vi "Initialize.vi"(8 "error in (no error)":errorcluster, 11 "State in":T1={"State"=enum."Idle", "Start Time"=timestamp(0 s since 1904-01-01), "Current Time"=timestamp(0 s since 1904-01-01), "First Iteration"=FALSE, "Data"={"D-O State"=enum."Off"}, "Process Name"="", "Output Error"=FALSE, "Log Started"=FALSE, "Cycle Period"=50.0, "Configuration"={"Valve Settings"={"D-O Settings"={"DAQmx Task Name"="", "Output Channel"=0, "Output Channel Names"=[], "Run?"=FALSE}, "VICI Electronic Actuator"={"VISA resource name"="", "Mode"=enum."Two Positions With Stops", "Simulated"=FALSE}}, "Valve Type"=enum."Digital Output Valve", "Time On (Sec)"=0.0, "Time Off (Sec)"=0.0}} {"Configuration"."Valve Settings"."D-O Settings"."Output Channel" items=["Choose a Channel"]}) -> (0 "error out":errorcluster, 1 "Initialized":bool, 3 "State out":T1={"State"=enum."Idle", "Start Time"=timestamp(0 s since 1904-01-01), "Current Time"=timestamp(0 s since 1904-01-01), "First Iteration"=FALSE, "Data"={"D-O State"=enum."Off"}, "Process Name"="", "Output Error"=FALSE, "Log Started"=FALSE, "Cycle Period"=50.0, "Configuration"={"Valve Settings"={"D-O Settings"={"DAQmx Task Name"="", "Output Channel"=0, "Output Channel Names"=[], "Run?"=FALSE}, "VICI Electronic Actuator"={"VISA resource name"="", "Mode"=enum."Two Positions With Stops", "Simulated"=FALSE}}, "Valve Type"=enum."Digital Output Valve", "Time On (Sec)"=0.0, "Time Off (Sec)"=0.0}} {"Configuration"."Valve Settings"."D-O Settings"."Output Channel" items=["Choose a Channel"]})   [LabVIEW 2018, in "D-O Module.lvlib" / "D-O Module Engine.lvlib"]
uses:
  D-O Module Engine.lvlib
  State Cluster.ctl
  State Enum.ctl
  Valve Clusters.ctl
  D-O Module Settings Cluster.ctl
  D-O Device Settings Cluster.ctl
  VICI Electronic Actuator/VICI Electronic Actuator Settings.ctl
  Tag VIs/Tag FGV Operation Enum.ctl
  Shared Variables/Dynamic Shared Variables.lvlib
  DIO Valve/VICI Electronic Actuator.lvlib
  D-O Module.lvlib
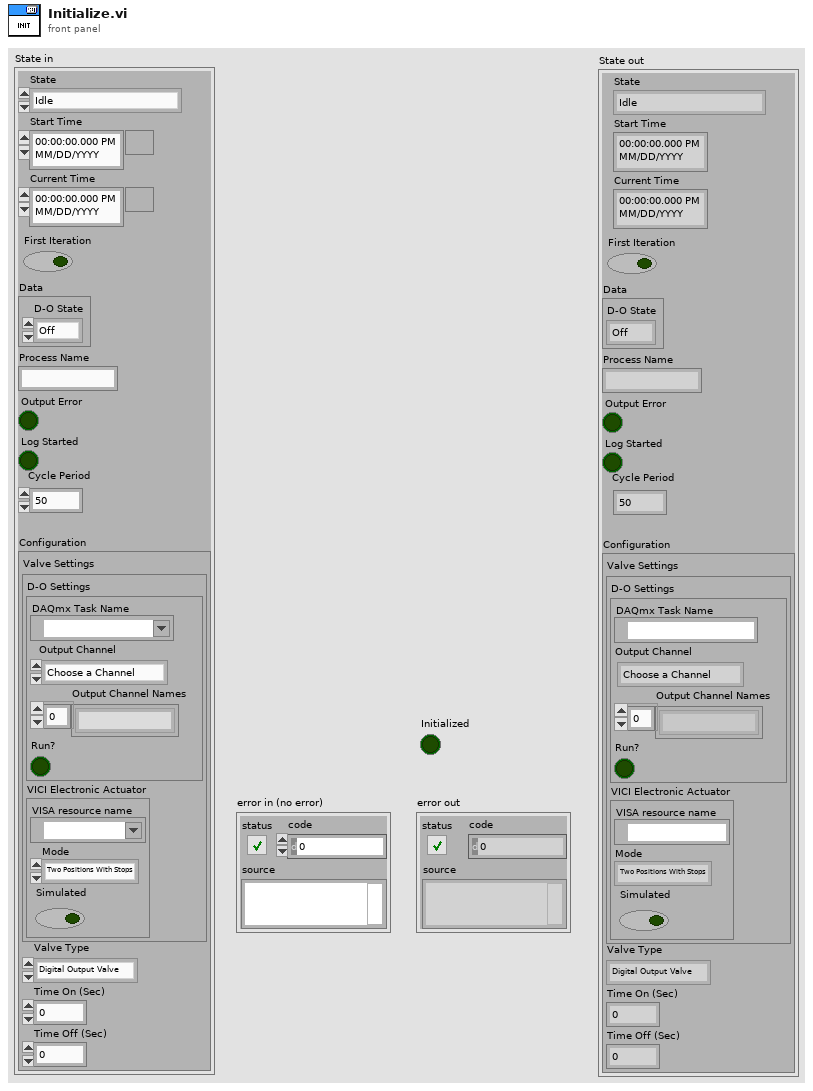
[diagram p1: front panel]
types:
  T1 = typedef "D-O Module.lvlib/D-O Module Engine.lvlib/State Cluster.ctl" = cluster{"State":T2, "Start Time":timestamp, "Current Time":timestamp, "First Iteration":bool, "Data":cluster{"D-O State":enum16{"Off", "On", "Not Initialized"}}, "Process Name":string, "Output Error":bool, "Log Started":bool, "Cycle Period":dbl, "Configuration":T3}
  T2 = typedef "D-O Module.lvlib/D-O Module Engine.lvlib/State Enum.ctl" = enum16{"Measuring", "Idle", "Paused"}
  T3 = typedef "D-O Module.lvlib/Valve Clusters.ctl" = cluster{"Valve Settings":T4, "Valve Type":enum16{"Digital Output Valve", "VICI Electronic Actuator"}, "Time On (Sec)":dbl, "Time Off (Sec)":dbl}
  T4 = typedef "D-O Module.lvlib/D-O Module Settings Cluster.ctl" = cluster{"D-O Settings":T5, "VICI Electronic Actuator":T6}
  T5 = typedef "D-O Module.lvlib/D-O Device Settings Cluster.ctl" = cluster{"DAQmx Task Name":refnum<k21>, "Output Channel":u16, "Output Channel Names":string[], "Run?":bool}
  T6 = typedef "VICI Electronic Actuator.lvlib/VICI Electronic Actuator Settings.ctl" = cluster{"VISA resource name":refnum<visa-resource-name>, "Mode":enum16{"Two Positions With Stops", "Two Positions Without Stops", "Mutiposition"}, "Simulated":bool}
  T7 = typedef "Tag FGV Operation Enum.ctl" = enum16{"Init", "Set Notification Queue", "Create Tag", "Commit", "Write Tag (Numeric)", "Write Tag (Boolean)", "Read All Tags", "Read One Tag", "Delete Tag Category", "Set Alarm Parameters (Numeric)", "Set Alarm Parameters (Boolean)", "Enable All Alarms", "Disable All Alarms", "Delete All Tags", "Read Alarms", "Ack Alarm"}
  T8 = enum16{"Digital Output Valve", "VICI Electronic Actuator"}
  T9 = typedef "D-O Module.lvlib/D-O Module Tag Names Cluster.ctl" = cluster{"D-O Status":string, "Output Device Tag":string}
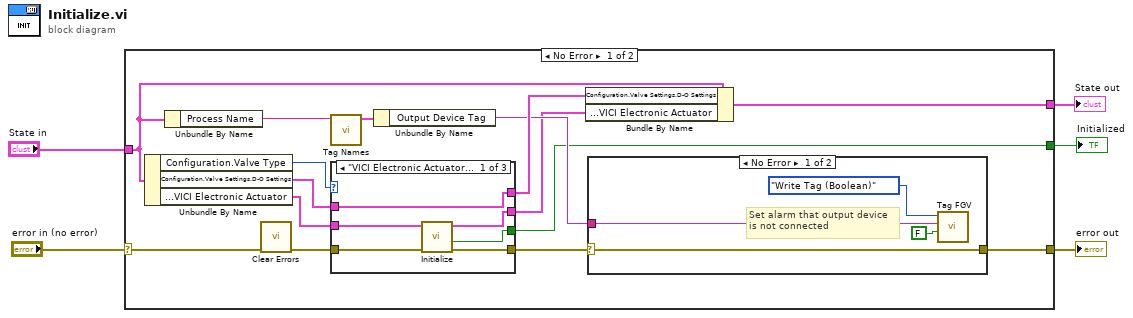
[diagram p0: block diagram]
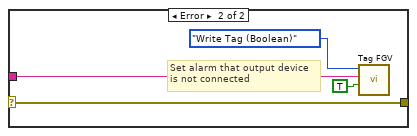
[diagram p2: hidden frame]
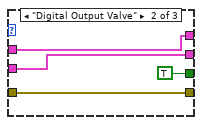
[diagram p3: hidden frame]
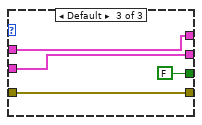
[diagram p4: hidden frame]
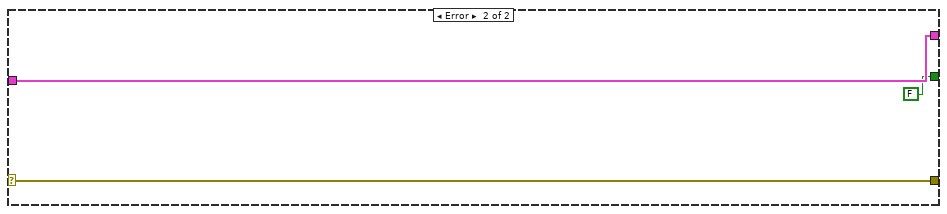
[diagram p5: hidden frame]
diagram:
  n1 = case shown="No Error" "error in (no error)" {
    selector: "error in (no error)" -> [w7 w45]
    tunnel: [w6 w45] -> w4
    tunnel: "State in" -> [w18 w44]
    tunnel: [w20 w44] -> w2
    tunnel: [w10 FALSE ("Initialized")] -> w1
    frame No Error {
      n2 = Unbundle By Name(w18) -> ("Configuration.Valve Type"=w11:T8, "Configuration.Valve Settings.D-O Settings"=w12:T5, "Configuration.Valve Settings.VICI Electronic Actuator"=w9:T6)
      n3 = Unbundle By Name(w18) -> ("Process Name"=w14:string)
      n4 = call <vilib>:"Clear Errors.vi"("error in (no error)"=w7) -> ("error out"=w17:errorcluster)  [unwired: 5 in, 1 out]
      n5 = call "Tag Names.vi"("Process Name"=w14) -> ("Pump Module Tag Names"=w13:T9)  [unwired: 8 in, 2 out]
      n6 = case shown="\"VICI Electronic Actuator\"" w11 {
        tunnel: w12 -> [w34 w38 w42]
        tunnel: [w34 w38 w42] -> w19
        tunnel: w17 -> [w30 w37 w41]
        tunnel: [w29 w37 w41] -> w16
        tunnel: [w31 TRUE ("Initialized") FALSE ("Initialized")] -> w10
        tunnel: w9 -> [w33 w35 w39]
        tunnel: [w32 w35 w39] -> w8
        frame "VICI Electronic Actuator" {
          n7 = call "Initialize.vi"("error in (no error)"=w30, "VICI Electronic Actuator"=w33) -> ("error out"=w29:errorcluster, "Initialized"=w31:bool, "VICI Electronic Actuator"=w32:T6)  [unwired: 6 in, 1 out]
        }
        frame "Digital Output Valve" {
        }
        frame Default {
        }
      }
      n8 = Unbundle By Name(w13) -> ("Output Device Tag"=w15:string)
      n9 = Bundle By Name(cluster=w18, "Configuration.Valve Settings.D-O Settings"=w19, "Configuration.Valve Settings.VICI Electronic Actuator"=w8) -> (w20:T1)
      n10 = case shown="No Error" w16 {
        selector: w16 -> [w24 w28]
        tunnel: [w24 w28] -> w6
        tunnel: w15 -> [w21 w27]
        frame No Error {
          # "Set alarm that output device\nis not connected"
          n11 = call "Tag FGV.vi"("Data"=FALSE, "Tag Name"=w21, "Operation"=Tag_FGV_Operation_Enum."Write Tag (Boolean)") -> ()  [unwired: 3 in, 6 out]
        }
        frame Error {
          # "Set alarm that output device\nis not connected"
          n12 = call "Tag FGV.vi"("Data"=TRUE, "Tag Name"=w27, "Operation"=Tag_FGV_Operation_Enum."Write Tag (Boolean)") -> ()  [unwired: 3 in, 6 out]
        }
      }
    }
    frame Error {
    }
  }
  "error out" <- w4
  "State out" <- w2
  "Initialized" <- w1
